vi "Read DIO Line.vi"(7 "DIO line":T1=1300 items=["FPGA LED"=6000, "Port3/DIO0"=1300, "Port3/DIO1"=1301, "Port3/DIO2"=1302, "Port3/DIO3"=1303, "Port3/DIO4"=1304, "Port3/DIO5"=1305, "Port3/DIO6"=1306, "Port3/DIO7"=1307, "Port3/DIO8"=1308, "Port3/DIO9"=1309], 8 "error in (no error)":errorcluster, 11 "starter kit host in":refnum<class "NI_Robotics_Starter Kit Host.lvclass">) -> (0 "error out":errorcluster, 2 "data":bool, 3 "starter kit host out":refnum<class "NI_Robotics_Starter Kit Host.lvclass">)   [LabVIEW 2017, in "NI_Robotics_Starter Kit Host.lvclass"]
doc: "Disables digital output and reads the value of a digital I/O line on the Starter Kit FPGA."
uses:
  <vilib>/robotics/Starter Kit/Host Interface/NI_Robotics_Starter Kit Host.lvclass
  <vilib>/robotics/Starter Kit/Direct IO/DIO Lines.ctl
  <vilib>/robotics/Starter Kit/Host Interface/NI_Robotics_Starter Kit Host.lvclass/NI_Robotics_Starter Kit Host.ctl
  <vilib>/robotics/Utilities/Generate Error.vi
  <vilib>/robotics/Starter Kit/Direct IO/NI_Robotics_Starter Kit Direct IO.lvclass
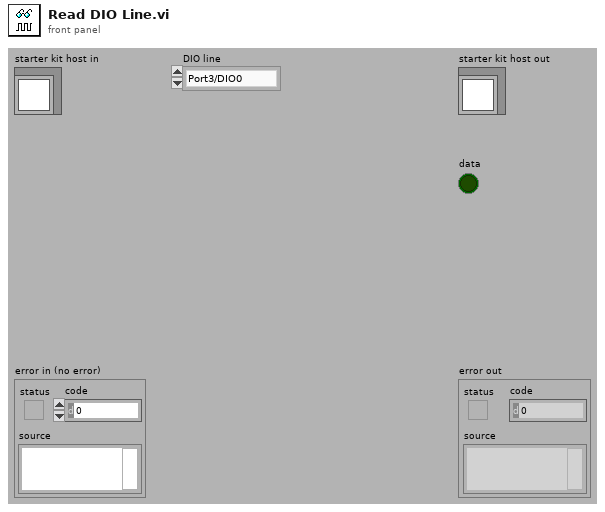
[diagram p1: front panel]
types:
  T1 = typedef "NI_Robotics_Starter Kit Direct IO.lvclass/DIO Lines.ctl" = u16
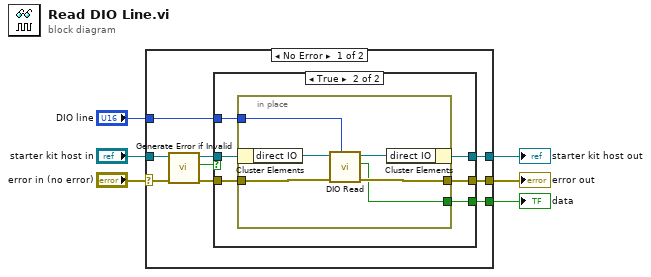
[diagram p0: block diagram]
diagram:
  n1 = case shown="No Error" "error in (no error)" {
    selector: "error in (no error)" -> [w9 w31]
    tunnel: [w13 w31] -> w5
    tunnel: [w15 w30] -> w3
    tunnel: "starter kit host in" -> [w11 w30]
    tunnel: "DIO line" -> [w14 _]
    tunnel: [w12 _] -> w1
    frame No Error {
      n2 = call <vilib>:"Generate Error if Invalid.vi"("error in (no error)"=w9, "starter kit host in"=w11) -> ("error out"=w8:errorcluster, "valid?"=w7:bool, "starter kit host out"=w10:refnum<class "NI_Robotics_Starter Kit Host.lvclass">)  [unwired: 7 in]
      n3 = case shown="True" w7 {
        tunnel: [w17 w23] -> w15
        tunnel: w14 -> [_ w22]
        tunnel: [w16 w21] -> w13
        tunnel: [_ w20] -> w12
        tunnel: w10 -> [w17 w19]
        tunnel: w8 -> [w16 w18]
        frame False {
        }
        frame True {
          n4 = in-place {
            in-place-border: w18 -> [w26]
            in-place-border: [w25] -> w21
            in-place-border: w22 -> [w27]
            in-place-border: [w24] -> w20
            n5 = in-place-cluster #1(w19) -> ("direct IO"=w29:refnum<class "NI_Robotics_Starter Kit Direct IO.lvclass">)
            n6 = call-dynamic "DIO Read.vi"("DIO line"=w27, "error in (no error)"=w26, "direct IO in"=w29) -> ("error out"=w25:errorcluster, "data"=w24:bool, "direct IO out"=w28:refnum<class "NI_Robotics_Starter Kit Direct IO.lvclass">)  [unwired: 6 in]
            n7 = in-place-cluster #1("direct IO"=w28) -> (w23:refnum<class "NI_Robotics_Starter Kit Host.lvclass">)
          }
        }
      }
    }
    frame Error {
    }
  }
  "error out" <- w5
  "starter kit host out" <- w3
  "data" <- w1
